vi "Database_User_Add.vi"(4 "error in":errorcluster, 5 "Language":T3, 6 "User Info":T2, 7 "connection reference":T1) -> (0 "error out":errorcluster, 1 "Message":string, 3 "connection reference out":T1)   [LabVIEW 2015]
uses:
  CustomControl/Lang_Control.ctl
  CustomControl/UserRight.ctl
  <vilib>/addons/database/Connection.llb/Conn ObjectReference.ctl
  <vilib>/addons/database/NI_Database_API.lvlib
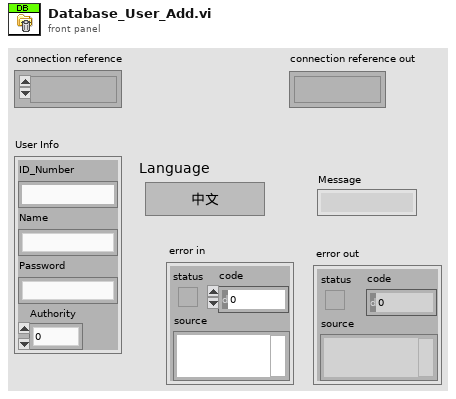
[diagram p1: front panel]
types:
  T1 = typedef "NI_Database_API.lvlib/Conn ObjectReference.ctl" = refnum<k1>
  T2 = typedef "UserRight.ctl" = cluster{"ID_Number":string, "Name":string, "Password":string, "Authority":i32}
  T3 = typedef "Lang_Control.ctl" = enum16{"中文", "English"}
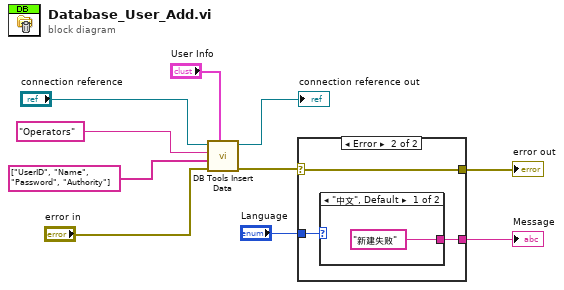
[diagram p0: block diagram]
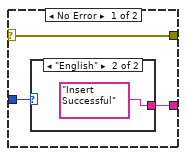
[diagram p2: hidden frame]
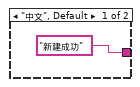
[diagram p3: hidden frame]
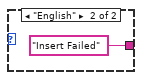
[diagram p4: hidden frame]
diagram:
  n1 = call <vilib>:"DB Tools Insert Data.vi"("data"="User Info", "error in (no error)"="error in", "columns"=string[] ["UserID", "Name", "Password", "Authority"], "table"="Operators", "connection reference"="connection reference") -> ("error out"=w2:errorcluster, "connection reference out"=→"connection reference out":T1)  [unwired: 5 in]
  n2 = case shown="Error" w2 {
    selector: w2 -> [w13 w18]
    tunnel: [w13 w18] -> w10
    tunnel: "Language" -> [w12 w17]
    tunnel: [w11 w16] -> w7
    frame No Error {
      n3 = case shown="\"English\"" w12 {
        tunnel: ["新建成功" "Insert Successful"] -> w11
        frame "中文", Default {
        }
        frame "English" {
        }
      }
    }
    frame Error {
      n4 = case shown="\"中文\", Default" w17 {
        tunnel: ["新建失败" "Insert Failed"] -> w16
        frame "中文", Default {
        }
        frame "English" {
        }
      }
    }
  }
  "error out" <- w10
  "Message" <- w7
